vi "commandInQueue.vi"(8 "error in (no error)":errorcluster, 11 "Monochromator in":refnum<class "Monochromator.lvclass">) -> (0 "error out":errorcluster, 2 "commandInQueue?":bool, 3 "Monochromator out":refnum<class "Monochromator.lvclass">)   [LabVIEW 2020, in "Monochromator.lvclass"]
uses:
  Monochromator.lvclass
  Monochromator.lvclass/Monochromator.ctl
  Commands/CommandQueue/CommandQueue.lvclass
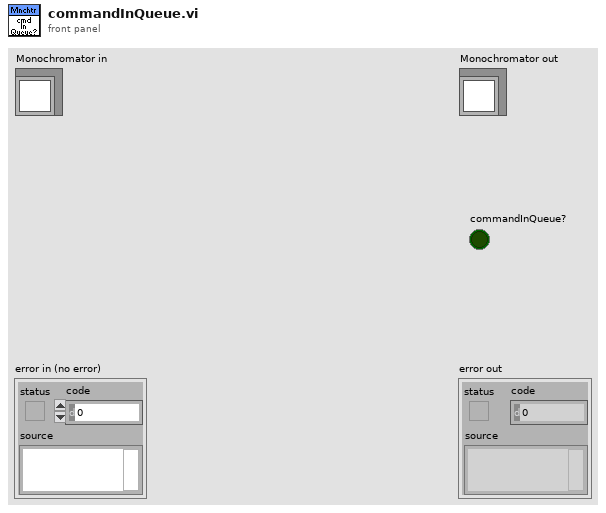
[diagram p1: front panel]
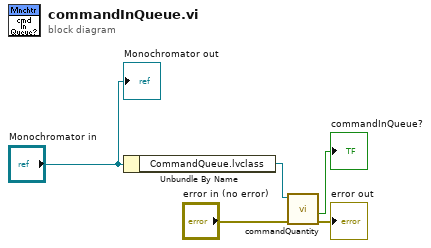
[diagram p0: block diagram]
diagram:
  n1 = Unbundle By Name("Monochromator in") -> ("CommandQueue.lvclass"=w4:refnum<class "CommandQueue.lvclass">)
  n2 = call "commandQuantity.vi"("error in (no error)"="error in (no error)", "CommandQueue in"=w4) -> ("error out"=→"error out":errorcluster, "x > 0?"=→"commandInQueue?":bool)  [unwired: 6 in, 2 out]
  "Monochromator out" <- "Monochromator in"
